vi "_EnumEditor_Interface.vi"(9 "EventsIn":T1, 10 "Events":T2) -> ()   [LabVIEW 2014, in "_EnumEditor.lvclass"]
uses:
  _EnumEditor.lvclass
  _EnumEditorVItypes.ctl
  GCMCore/Providers/Veritech_GCM/Support/Framework/_Plugins/_LVCMPlugin/GCMPlugin_EventsOut.ctl
  GCMCore/Providers/Veritech_GCM/Support/Framework/_Plugins/_LVCMPlugin/GCMPlugin_EventsIn.ctl
  _EnumEditorStates.ctl
  _EnumEditor.lvclass/_EnumEditor.ctl
  <vilib>/event_ctls.llb/eventvkey.ctl
  _EnumEditor_GetVIref.vi
  _EnumEditor_SetVIref.vi
  _EnumEditor_SetActualStrings.vi
  _EnumEditor_SetInitialStrings.vi
  _EnumEditor_SetEnumRef.vi
  _EnumEditor_SetVI_Type.vi
  _EnumEditor_GetActualStrings.vi
  _EnumEditor_GetVI_Type.vi
  _EnumEditor_GetEnumRef.vi
  _EnumEditor_GetInitialStrings.vi
  GCMCore/Providers/Veritech_GCM/Support/Framework/_Plugins/GCMPlugin/GCMPlugin.lvclass
panel:
  in  "Cancel":bool
  in  "Save":bool
  in  "EnumType":T3
  in  "EnumStates":i32(listbox)
  # "Warning!\nIf you change enum with typedef\non control, you disconnect all instances, \nand can't back this operation."
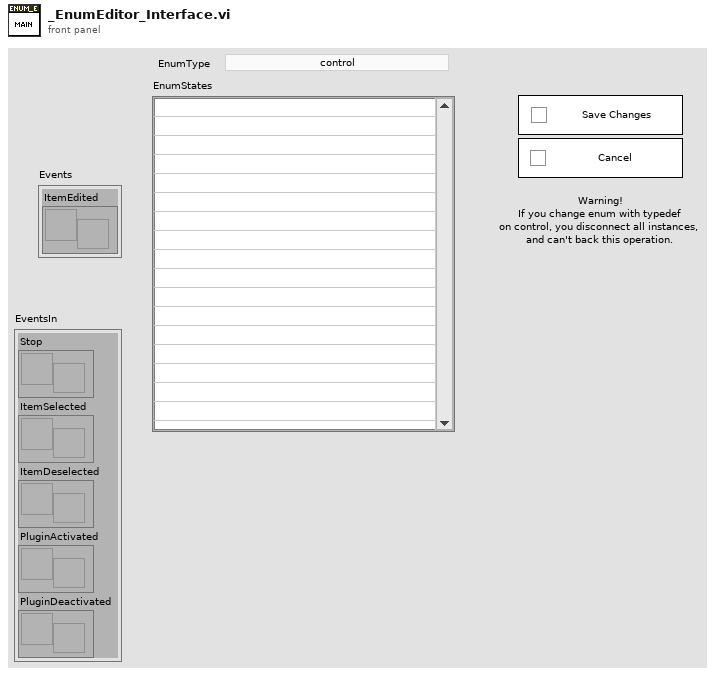
[diagram p1: front panel]
types:
  T1 = typedef "GCMPlugin.lvclass/GCMPlugin_EventsIn.ctl" = cluster{"Stop":refnum<user-event>, "ItemSelected":refnum<user-event>, "ItemDeselected":refnum<user-event>, "PluginActivated":refnum<user-event>, "PluginDeactivated":refnum<user-event>}
  T2 = typedef "GCMPlugin.lvclass/GCMPlugin_EventsOut.ctl" = cluster{"ItemEdited":refnum<user-event>}
  T3 = typedef "_EnumEditor.lvclass/_EnumEditorVItypes.ctl" = enum32{"control", "typedef", "strict typedef"}
  T4 = typedef "_EnumEditor.lvclass/_EnumEditorStates.ctl" = enum16{"Init", "WaitForEvent", "Save", "Cancel", "SetControls"}
  T5 = typedef "eventvkey.ctl" = enum16{"ASCII", "Enter", "Return", "Shift", "Ctrl", "Alt", "Cmd", "Opt", "Caps", "NumLock", "Clear", "Break", "Up", "Down", "Left", "Right", "Insert", "Delete", "Home", "End", "PageUp", "PageDown", "Escape", "Help", "Pause", "ScrollLock", "F1", "F2", "F3", "F4", "F5", "F6", "F7", "F8", "F9", "F10", "F11", "F12", "F13", "F14", "F15", "F16", "F17", "F18", "F19", "F20", "F21", "F22", "F23", "F24", "Play", "VolumeUp", "VolumeDown", "Mute", "Two Byte Char"}
  T6 = enum32{"not a control VI", "control", "typedef", "strict typedef"}
  T7 = typedef "LVPoint32TypeDef.ctl" = cluster{"Horizontal":i32, "Vertical":i32}
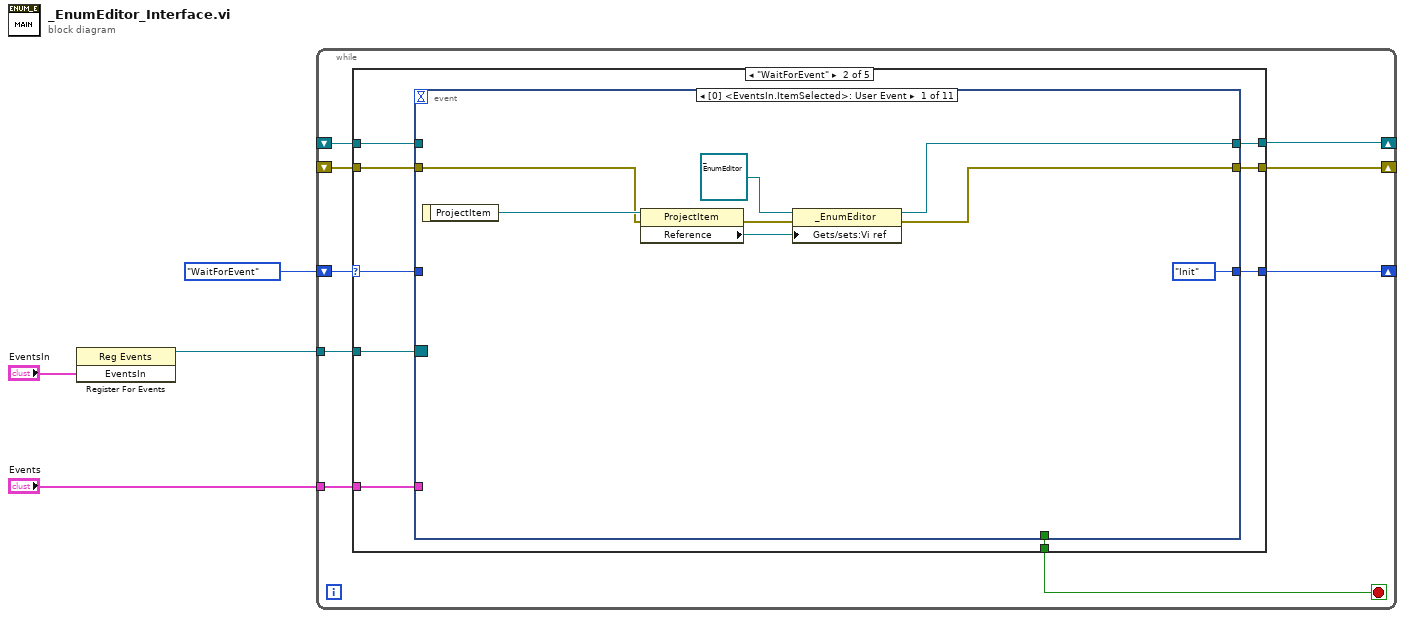
[diagram p0: block diagram]
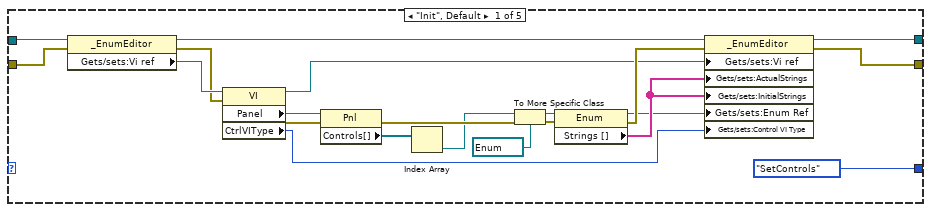
[diagram p2: hidden frame]
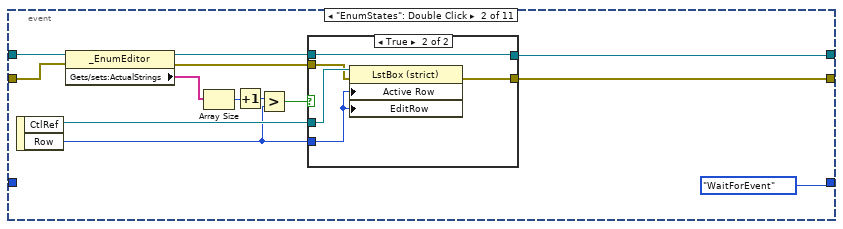
[diagram p3: hidden frame]
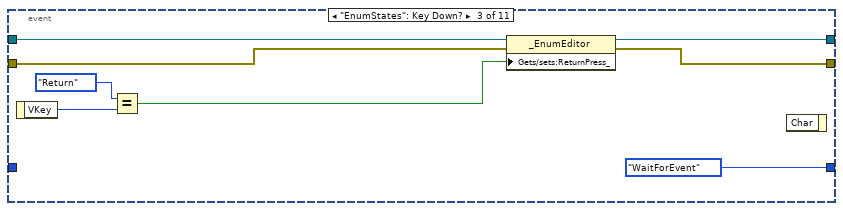
[diagram p5: hidden frame]
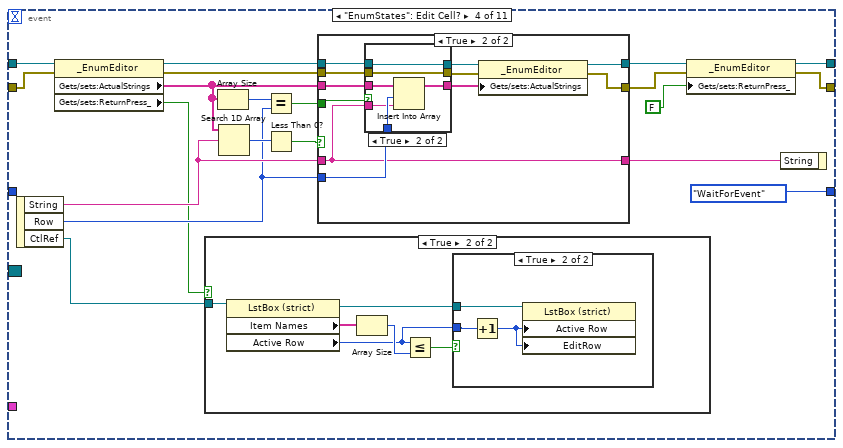
[diagram p6: hidden frame]
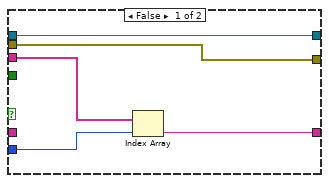
[diagram p9: hidden frame]
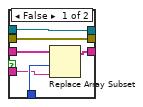
[diagram p10: hidden frame]
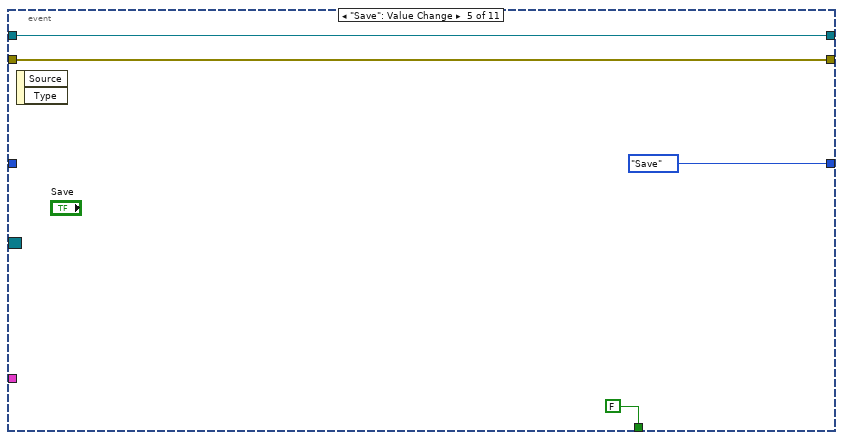
[diagram p11: hidden frame]
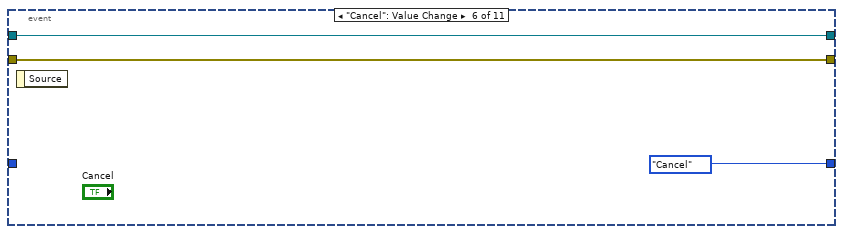
[diagram p12: hidden frame]
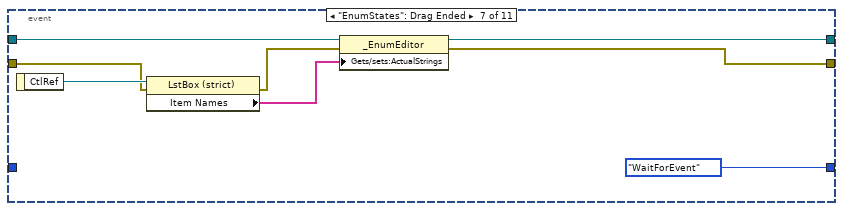
[diagram p13: hidden frame]
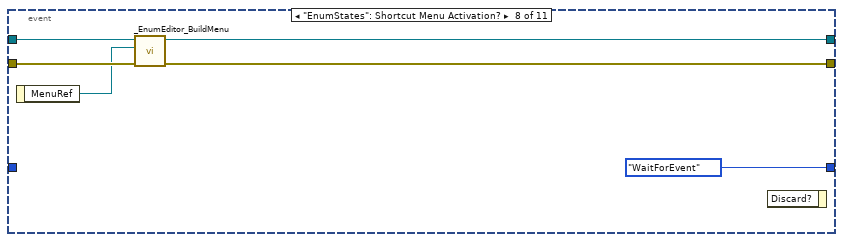
[diagram p14: hidden frame]
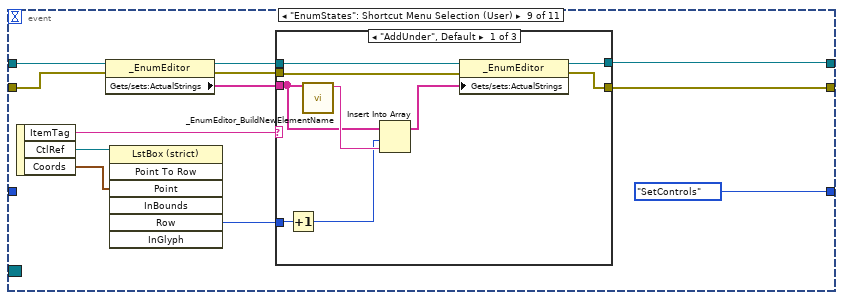
[diagram p15: hidden frame]
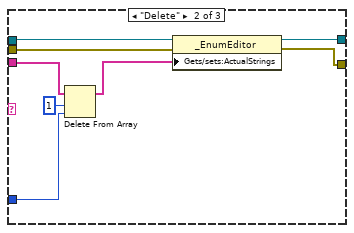
[diagram p16: hidden frame]
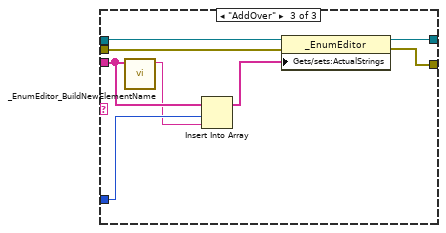
[diagram p17: hidden frame]
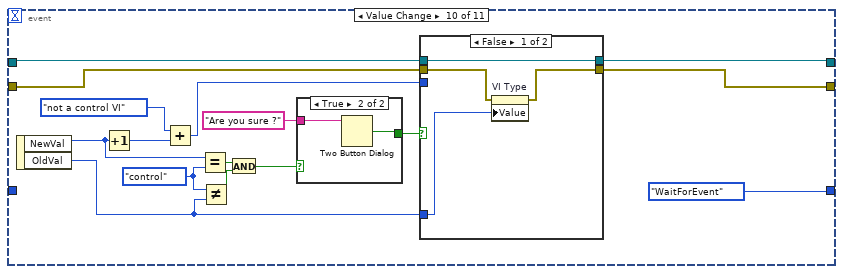
[diagram p18: hidden frame]
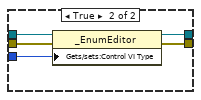
[diagram p19: hidden frame]
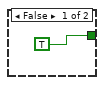
[diagram p20: hidden frame]
diagram:
  n1 = register-events("EventsIn") -> (reference out=w1:refnum<event-registration>)  [unwired: 2 in, 1 out]
  n2 = while {
    shift-right: [w7] -> _
    shift-left: _ -> [w11]
    shift-right: [w10] -> _
    shift-left: _ -> [w12]
    shift-right: [w9] -> _
    shift-left: _EnumEditorStates."WaitForEvent" -> [w13]
    tunnel: "Events" -> [w6]
    tunnel: w1 -> [w5]
    stop <- w8 stop-if-true
    n3 = case shown="\"WaitForEvent\"" w13 {
      selector: w13 -> [_ w38 _ _ _]
      tunnel: w12 -> [w26 w43 w239 w247 w255]
      tunnel: w11 -> [w25 w42 w238 w246 w254]
      tunnel: [w19 w41 w237 w242 w259] -> w10
      tunnel: [w18 w40 w229 w241 w256] -> w7
      tunnel: [_EnumEditorStates."SetControls" w39 _EnumEditorStates."Init" _EnumEditorStates."Init" _EnumEditorStates."WaitForEvent"] -> w9
      tunnel: [_ w37 _ _ _] -> w8
      tunnel: w6 -> [_ w36 _ _ _]
      tunnel: w5 -> [_ w35 _ _ _]
      frame "Init", Default {
        n4 = property class="_EnumEditor"(reference=w26, error in=w25) -> (reference out=w22:refnum<class "_EnumEditor.lvclass">, error out=w23:errorcluster, "Gets/sets:Vi ref"=w24:refnum<vi>)
        n5 = property class="VI"(reference=w24, error in=w23) -> (reference out=w20:refnum<vi>, error out=w32:errorcluster, "Panel"=w34:refnum<vi>, "CtrlVIType"=w14:T6)
        n6 = property class="Pnl"(reference=w34, error in=w32) -> (error out=w31:errorcluster, "Controls[]"=w33:refnum<vi>[])  [unwired: 1 out]
        n7 = Index Array(array=w33) -> (element=w30:refnum<vi>)  [unwired: 1 in]
        n8 = To More Specific Class(target class=refnum<vi> refnum ("reference"), reference=w30, error in=w31) -> (specific class reference=w28:refnum<vi>, error out=w27:errorcluster)
        n9 = property class="Enum"(reference=w28, error in=w27) -> (reference out=w15:refnum<vi>, error out=w21:errorcluster, "Strings []"=w16:string[])
        n10 = property class="_EnumEditor"(reference=w22, error in=w21, "Gets/sets:Vi ref"=w20, "Gets/sets:ActualStrings"=w16, "Gets/sets:InitialStrings"=w16, "Gets/sets:Enum Ref"=w15, "Gets/sets:Control VI Type"=w14) -> (reference out=w19:refnum<class "_EnumEditor.lvclass">, error out=w18:errorcluster)
      }
      frame "WaitForEvent" {
        n11 = event shown="[0] <EventsIn.ItemSelected>: User Event" {
          selector: w35 -> [_ _ _ _ _ _ _ _ _ _ _]
          dyn-events: _ -> [_ _ _ _ _ _ _ _ _ _ _]
          timeout: _ -> [_ _ _ _ _ _ _ _ _ _ _]
          tunnel: w43 -> [_ w61 w76 w99 w138 w142 w150 w157 w165 w210 w226]
          tunnel: w42 -> [w48 w60 w74 w98 w137 w141 w148 w156 w164 w209 w225]
          tunnel: [w46 w63 w75 w82 w138 w142 w145 w154 w160 w208 w226] -> w41
          tunnel: [w47 w62 w73 w84 w137 w141 w144 w153 w159 w207 w225] -> w40
          tunnel: [_EnumEditorStates."Init" _EnumEditorStates."WaitForEvent" _EnumEditorStates."WaitForEvent" _EnumEditorStates."WaitForEvent" _EnumEditorStates."Save" _EnumEditorStates."Cancel" _EnumEditorStates."WaitForEvent" _EnumEditorStates."WaitForEvent" _EnumEditorStates."SetControls" _EnumEditorStates."WaitForEvent" _EnumEditorStates."WaitForEvent"] -> w39
          tunnel: w38 -> [_ _ _ _ _ _ _ _ _ _ _]
          tunnel: [_ _ _ _ FALSE _ _ _ _ _ TRUE] -> w37
          tunnel: w36 -> [_ _ _ _ _ _ _ _ _ _ _]
          event User Event {
            n12 = event-data() -> ("ProjectItem"=w49:refnum<vi>)  [unwired: 1 in]
            n13 = property class="ProjectItem"(reference=w49, error in=w48) -> (error out=w51:errorcluster, "Reference"=w44:refnum<vi>)  [unwired: 1 out]
            n14 = property class="_EnumEditor"(reference=refnum<class "_EnumEditor.lvclass"> refnum ("_EnumEditor.lvclass"), error in=w51, "Gets/sets:Vi ref"=w44) -> (reference out=w46:refnum<class "_EnumEditor.lvclass">, error out=w47:errorcluster)
          }
          event "EnumStates": Double Click {
            n15 = event-data() -> ("CtlRef"=w64:refnum<vi>, "Row"=w58:i32)  [unwired: 1 in]
            n16 = property class="_EnumEditor"(reference=w61, error in=w60) -> (reference out=w57:refnum<class "_EnumEditor.lvclass">, error out=w56:errorcluster, "Gets/sets:ActualStrings"=w59:string[])
            n17 = Array Size(array=w59) -> (size(s)=w54:i32)
            n18 = Increment(x=w54) -> (x+1=w53:i32)
            n19 = Greater?(x=w53, y=w58) -> (0:w55:bool)
            n20 = case shown="True" w55 {
              tunnel: w64 -> [_ w71]
              tunnel: w58 -> [_ w69]
              tunnel: [w66 w68] -> w63
              tunnel: [w65 w70] -> w62
              tunnel: w57 -> [w66 w68]
              tunnel: w56 -> [w65 w67]
              frame False {
              }
              frame True {
                n21 = property class="LstBox (strict)"(reference=w71, error in=w67, "Active Row"=w69, "EditRow"=w69) -> (error out=w70:errorcluster)  [unwired: 1 out]
              }
            }
          }
          event "EnumStates": Key Down? {
            n22 = event-data() -> ("VKey"=w79:T5)  [unwired: 1 in]
            n23 = Equal?(x=eventvkey."Return" ("VKey"), y=w79) -> (x = y?=w72:bool)
            n24 = property class="_EnumEditor"(reference=w76, error in=w74, "Gets/sets:ReturnPress_"=w72) -> (reference out=w75:refnum<class "_EnumEditor.lvclass">, error out=w73:errorcluster)
            n25 = event-data() -> ()  [unwired: 2 in, 1 out]
          }
          event "EnumStates": Edit Cell? {
            n26 = event-data() -> ("String"=w91:string, "Row"=w89:i32, "CtlRef"=w85:refnum<vi>)  [unwired: 1 in]
            n27 = property class="_EnumEditor"(reference=w99, error in=w98) -> (reference out=w94:refnum<class "_EnumEditor.lvclass">, error out=w92:errorcluster, "Gets/sets:ActualStrings"=w88:string[], "Gets/sets:ReturnPress_"=w80:bool)
            n28 = case shown="True" w80 {
              tunnel: w85 -> [_ w105]
              frame False {
              }
              frame True {
                n29 = property class="LstBox (strict)"(reference=w105) -> (reference out=w102:refnum<vi>, "Item Names"=w104:string[], "Active Row"=w100:i32)  [unwired: 1 in, 1 out]
                n30 = Array Size(array=w104) -> (size(s)=w103:i32)
                n31 = Less Or Equal?(x=w100, y=w103) -> (x <= y?=w101:bool)
                n32 = case shown="True" w101 {
                  tunnel: w102 -> [_ w108]
                  tunnel: w100 -> [_ w107]
                  frame False {
                  }
                  frame True {
                    n33 = Increment(x=w107) -> (x+1=w106:i32)
                    n34 = property class="LstBox (strict)"(reference=w108, "Active Row"=w106, "EditRow"=w106) -> ()  [unwired: 1 in, 2 out]
                  }
                }
              }
            }
            n35 = Array Size(array=w88) -> (size(s)=w87:i32)
            n36 = Search 1D Array(1D array=w88, element=w91) -> (index of element=w97:i32)  [unwired: 1 in]
            n37 = Equal?(x=w87, y=w89) -> (x = y?=w86:bool)
            n38 = Less Than 0?(x=w97) -> (x < 0?=w96:bool)
            n39 = case shown="True" w96 {
              tunnel: w88 -> [w113 w124]
              tunnel: w89 -> [w112 w123]
              tunnel: [w111 w122] -> w95
              tunnel: [w110 w121] -> w83
              tunnel: w94 -> [w110 w114]
              tunnel: [w109 w120] -> w93
              tunnel: w92 -> [w109 w116]
              tunnel: w91 -> [_ w122]
              tunnel: w86 -> [_ w118]
              frame False {
                n40 = Index Array(array=w113, index=w112) -> (element=w111:string)
              }
              frame True {
                n41 = case shown="True" w118 {
                  tunnel: w124 -> [w130 w136]
                  tunnel: w123 -> [w129 w134]
                  tunnel: w122 -> [w128 w133]
                  tunnel: [w127 w135] -> w119
                  tunnel: [w126 w131] -> w117
                  tunnel: w116 -> [w126 w131]
                  tunnel: [w125 w132] -> w115
                  tunnel: w114 -> [w125 w132]
                  frame False {
                    n42 = Replace Array Subset(array=w130, new element=w128, index=w129) -> (w127:string[])
                  }
                  frame True {
                    n43 = Insert Into Array(array=w136, index=w134, new element=w133) -> (w135:string[])
                  }
                }
                n44 = property class="_EnumEditor"(reference=w115, error in=w117, "Gets/sets:ActualStrings"=w119) -> (reference out=w121:refnum<class "_EnumEditor.lvclass">, error out=w120:errorcluster)
              }
            }
            n45 = property class="_EnumEditor"(reference=w83, error in=w93, "Gets/sets:ReturnPress_"=FALSE ("ReturnPress_")) -> (reference out=w82:refnum<class "_EnumEditor.lvclass">, error out=w84:errorcluster)
            n46 = event-data("String"=w95) -> ()  [unwired: 1 in, 1 out]
          }
          event "Save": Value Change {
            n47 = event-data() -> ()  [unwired: 1 in, 2 out]
          }
          event "Cancel": Value Change {
            n48 = event-data() -> ()  [unwired: 1 in, 1 out]
          }
          event "EnumStates": Drag Ended {
            n49 = event-data() -> ("CtlRef"=w149:refnum<vi>)  [unwired: 1 in]
            n50 = property class="LstBox (strict)"(reference=w149, error in=w148) -> (error out=w147:errorcluster, "Item Names"=w146:string[])  [unwired: 1 out]
            n51 = property class="_EnumEditor"(reference=w150, error in=w147, "Gets/sets:ActualStrings"=w146) -> (reference out=w145:refnum<class "_EnumEditor.lvclass">, error out=w144:errorcluster)
          }
          event "EnumStates": Shortcut Menu Activation? {
            n52 = event-data() -> ("MenuRef"=w155:refnum<k9>)  [unwired: 1 in]
            n53 = call "_EnumEditor_BuildMenu.vi"("error in (no error)"=w156, "menu reference"=w155, "_EnumEditor in"=w157) -> ("error out"=w153:errorcluster, "_EnumEditor out"=w154:refnum<class "_EnumEditor.lvclass">)  [unwired: 7 in]
            n54 = event-data() -> ()  [unwired: 2 in, 1 out]
          }
          event "EnumStates": Shortcut Menu Selection (User) {
            n55 = event-data() -> ("ItemTag"=w167:string, "CtlRef"=w169:refnum<vi>, "Coords"=w168:T7)  [unwired: 1 in]
            n56 = property class="_EnumEditor"(reference=w165, error in=w164) -> (reference out=w163:refnum<class "_EnumEditor.lvclass">, error out=w162:errorcluster, "Gets/sets:ActualStrings"=w161:string[])
            n57 = invoke class="LstBox (strict)" method="Point To Row"(reference=w169, "Point"=w168) -> ("Row"=w166:i32)  [unwired: 5 in, 6 out]
            n58 = case shown="\"AddUnder\", Default" w167 {
              tunnel: w166 -> [w171 w181 w194]
              tunnel: w163 -> [w176 w186 w191]
              tunnel: w162 -> [w175 w185 w190]
              tunnel: w161 -> [w172 w182 w193]
              tunnel: [w173 w184 w188] -> w160
              tunnel: [w174 w183 w187] -> w159
              frame "AddUnder", Default {
                n59 = Increment(x=w171) -> (x+1=w170:i32)
                n60 = call "_EnumEditor_BuildNewElementName.vi"("ActualStrings"=w172) -> ("New string"=w178:string)  [unwired: 10 in]
                n61 = Insert Into Array(array=w172, index=w170, new element=w178) -> (w177:string[])
                n62 = property class="_EnumEditor"(reference=w176, error in=w175, "Gets/sets:ActualStrings"=w177) -> (reference out=w173:refnum<class "_EnumEditor.lvclass">, error out=w174:errorcluster)
              }
              frame "Delete" {
                n63 = Delete From Array(array=w182, length=1, index=w181) -> (array with subset deleted=w179:string[])  [unwired: 1 out]
                n64 = property class="_EnumEditor"(reference=w186, error in=w185, "Gets/sets:ActualStrings"=w179) -> (reference out=w184:refnum<class "_EnumEditor.lvclass">, error out=w183:errorcluster)
              }
              frame "AddOver" {
                n65 = call "_EnumEditor_BuildNewElementName.vi"("ActualStrings"=w193) -> ("New string"=w192:string)  [unwired: 10 in]
                n66 = Insert Into Array(array=w193, index=w194, new element=w192) -> (w189:string[])
                n67 = property class="_EnumEditor"(reference=w191, error in=w190, "Gets/sets:ActualStrings"=w189) -> (reference out=w188:refnum<class "_EnumEditor.lvclass">, error out=w187:errorcluster)
              }
            }
          }
          event Value Change {
            w201 = _EnumEditorVItypes."control" ("NewVal")
            n68 = event-data() -> ("NewVal"=w202:T3, "OldVal"=w195:T3)  [unwired: 1 in]
            n69 = Increment(x=w202) -> (x+1=w203:T3)
            n70 = Add(x=T6."not a control VI" ("Control VI Type"), y=w203) -> (x+y=w204:u32)
            n71 = Equal?(x=w202, y=w201) -> (x = y?=w200:bool)
            n72 = Not Equal?(x=w201, y=w195) -> (x != y?=w199:bool)
            n73 = And(x=w200, y=w199) -> (x .and. y?=w198:bool)
            n74 = case shown="True" w198 {
              tunnel: [TRUE w222] -> w197
              tunnel: "Are you sure ?" ("message") -> [_ w221]
              frame False {
              }
              frame True {
                n75 = Two Button Dialog(message=w221) -> (T button?=w222:bool)  [unwired: 2 in]
              }
            }
            n76 = case shown="False" w197 {
              tunnel: w210 -> [w214 w219]
              tunnel: w209 -> [w213 w218]
              tunnel: [w214 w217] -> w208
              tunnel: [w212 w216] -> w207
              tunnel: w204 -> [_ w215]
              tunnel: w195 -> [w211 _]
              frame False {
                n77 = property on="VI Type" class="Enum (strict)"(error in=w213, "Value"=w211) -> (error out=w212:errorcluster)  [unwired: 1 in, 1 out]
              }
              frame True {
                n78 = property class="_EnumEditor"(reference=w219, error in=w218, "Gets/sets:Control VI Type"=w215) -> (reference out=w217:refnum<class "_EnumEditor.lvclass">, error out=w216:errorcluster)
              }
            }
          }
          event User Event {
            n79 = event-data() -> ()  [unwired: 1 in, 1 out]
          }
        }
      }
      frame "Save" {
        n80 = property class="_EnumEditor"(reference=w239, error in=w238) -> (reference out=w237:refnum<class "_EnumEditor.lvclass">, error out=w234:errorcluster, "Gets/sets:Vi ref"=w228:refnum<vi>, "Gets/sets:Control VI Type"=w227:T6, "Gets/sets:Enum Ref"=w236:refnum<vi>, "Gets/sets:ActualStrings"=w235:string[])
        n81 = property class="Enum"(reference=w236, error in=w234, "Strings []"=w235) -> (error out=w233:errorcluster)  [unwired: 1 out]
        n82 = property class="VI"(reference=w228, error in=w233, "CtrlVIType"=w227) -> (reference out=w232:refnum<vi>, error out=w230:errorcluster, "Path"=w231:path)
        n83 = invoke class="VI" method="Save.For Previous"(reference=w232, error in=w230, "Path to saved file"=w231) -> (error out=w229:errorcluster)  [unwired: 3 in, 5 out]
      }
      frame "Cancel" {
        n84 = property class="_EnumEditor"(reference=w247, error in=w246) -> (reference out=w245:refnum<class "_EnumEditor.lvclass">, error out=w243:errorcluster, "Gets/sets:InitialStrings"=w244:string[])
        n85 = property class="_EnumEditor"(reference=w245, error in=w243, "Gets/sets:ActualStrings"=w244) -> (reference out=w242:refnum<class "_EnumEditor.lvclass">, error out=w241:errorcluster)
      }
      frame "SetControls" {
        n86 = call "_EnumEditor_CheckUnique.vi"("error in (no error)"=w254, "_EnumEditor in"=w255) -> ("error out"=w252:errorcluster, "_EnumEditor out"=w253:refnum<class "_EnumEditor.lvclass">)  [unwired: 8 in]
        n87 = property class="_EnumEditor"(reference=w253, error in=w252) -> (reference out=w259:refnum<class "_EnumEditor.lvclass">, error out=w261:errorcluster, "Gets/sets:ActualStrings"=w260:string[], "Gets/sets:Control VI Type"=w251:T6)
        n88 = To Unsigned Long Integer(number=w251) -> (unsigned 32bit integer=w250:u32)
        n89 = Decrement(x=w250) -> (x-1=w249:u32)
        n90 = property on="EnumStates" class="LstBox (strict)"(error in=w261, "Item Names"=w260) -> (error out=w257:errorcluster)  [unwired: 1 in, 1 out]
        n91 = property on="VI Type" class="Enum (strict)"(error in=w257, "Value"=w249) -> (error out=w256:errorcluster)  [unwired: 1 in, 1 out]
      }
    }
  }
